vi "Parallel edge distance.vi"(2 "Edge 2 start point":sgl[](array[numeric]), 3 "Edge 2 (not unit)":sgl[](array[numeric]), 4 "Edge 1 start point":sgl[](array[numeric]), 5 "Edge 1 (not unit)":sgl[](array[numeric])) -> (0 "Distance vector":sgl[](array[numeric]), 1 "Projections overlap":bool)   [LabVIEW 2014]
panel:
  # "PN 13/01/2015"
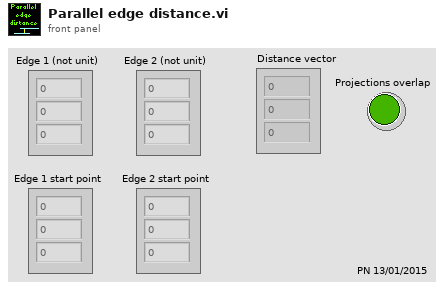
[diagram p1: front panel]
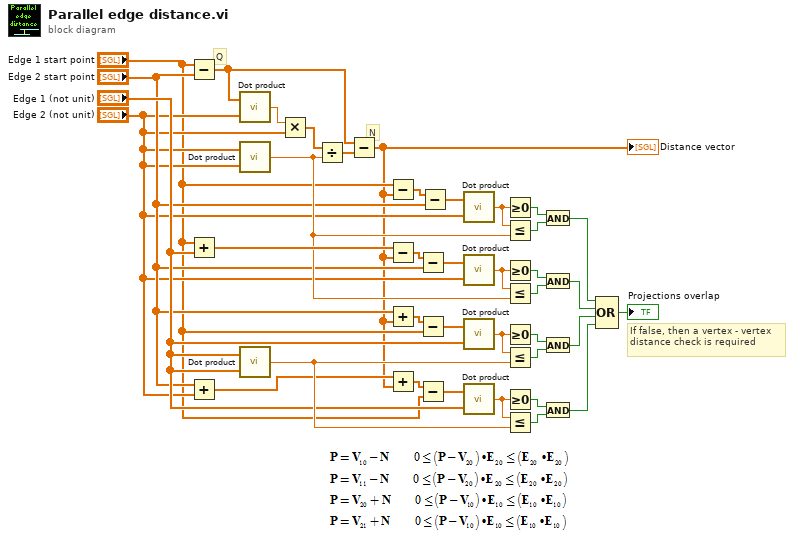
[diagram p0: block diagram]
diagram:
  # "If false, then a vertex - vertex distance check is required"
  # "N"
  # "Q"
  n1 = Subtract(x="Edge 1 start point", y="Edge 2 start point") -> (x-y=w36:sgl[])
  n2 = Add(x="Edge 1 start point", y="Edge 1 (not unit)") -> (x+y=w28:sgl[])
  n3 = Add(x="Edge 2 start point", y="Edge 2 (not unit)") -> (x+y=w8:sgl[])
  n4 = call "Dot product.vi"("B"="Edge 2 (not unit)", "A"=w36) -> ("A . B"=w38:sgl)
  n5 = call "Dot product.vi"("B"="Edge 2 (not unit)", "A"="Edge 2 (not unit)") -> ("A . B"=w27:sgl)
  n6 = call "Dot product.vi"("B"="Edge 1 (not unit)", "A"="Edge 1 (not unit)") -> ("A . B"=w12:sgl)
  n7 = Multiply(x=w38, y="Edge 2 (not unit)") -> (x*y=w37:sgl[])
  n8 = Divide(x=w37, y=w27) -> (x/y=w35:sgl[])
  n9 = Subtract(x=w36, y=w35) -> (x-y=w2:sgl[])
  "Distance vector" <- w2
  n10 = Subtract(x="Edge 1 start point", y=w2) -> (x-y=w26:sgl[])
  n11 = Subtract(x=w28, y=w2) -> (x-y=w24:sgl[])
  n12 = Add(x="Edge 2 start point", y=w2) -> (x+y=w21:sgl[])
  n13 = Add(x=w8, y=w2) -> (x+y=w14:sgl[])
  n14 = Subtract(x=w24, y="Edge 2 start point") -> (x-y=w23:sgl[])
  n15 = Subtract(x=w21, y="Edge 1 start point") -> (x-y=w22:sgl[])
  n16 = Subtract(x=w14, y="Edge 1 start point") -> (x-y=w13:sgl[])
  n17 = Subtract(x=w26, y="Edge 2 start point") -> (x-y=w25:sgl[])
  n18 = call "Dot product.vi"("B"="Edge 2 (not unit)", "A"=w25) -> ("A . B"=w34:sgl)
  n19 = call "Dot product.vi"("B"="Edge 2 (not unit)", "A"=w23) -> ("A . B"=w29:sgl)
  n20 = call "Dot product.vi"("B"="Edge 1 (not unit)", "A"=w22) -> ("A . B"=w20:sgl)
  n21 = call "Dot product.vi"("B"="Edge 1 (not unit)", "A"=w13) -> ("A . B"=w15:sgl)
  n22 = Greater Or Equal To 0?(x=w34) -> (x >= 0?=w33:bool)
  n23 = Less Or Equal?(x=w34, y=w27) -> (x <= y?=w32:bool)
  n24 = Greater Or Equal To 0?(x=w29) -> (x >= 0?=w30:bool)
  n25 = Less Or Equal?(x=w29, y=w27) -> (x <= y?=w31:bool)
  n26 = Greater Or Equal To 0?(x=w20) -> (x >= 0?=w19:bool)
  n27 = Less Or Equal?(x=w20, y=w12) -> (x <= y?=w18:bool)
  n28 = Greater Or Equal To 0?(x=w15) -> (x >= 0?=w16:bool)
  n29 = Less Or Equal?(x=w15, y=w12) -> (x <= y?=w17:bool)
  n30 = And(x=w33, y=w32) -> (x .and. y?=w6:bool)
  n31 = And(x=w30, y=w31) -> (x .and. y?=w5:bool)
  n32 = And(x=w19, y=w18) -> (x .and. y?=w4:bool)
  n33 = And(x=w16, y=w17) -> (x .and. y?=w3:bool)
  n34 = Compound Arithmetic op=OR(w6, w5, w4, w3) -> (→"Projections overlap":bool)
